vi "WPI_RobotDriveOpen2MotorWithVictor.vi"(4 "InverseTransformVIRef":T1, 5 "Right Motor Inverted":bool, 6 "TransformVIRef":T1, 7 "Left Motor Inverted":bool, 8 "error in (no error)":errorcluster, 10 "Right Motor":T5=enum."Invalid", 11 "Left Motor":T5=enum."Invalid") -> (0 "error out":errorcluster, 3 "RobotDriveDevRef":T2={"DevStatus"={"status"=FALSE, "code"=0, "source"=""}, "Motors[]"=[], "Square Inputs"=FALSE, "Max Output"=1.0, "Isochronous"=FALSE})   [LabVIEW 2011]
doc: "Opens a reference to the robot drive for a two-motor robot using Victor motor controllers.\n\nThis software is licensed. Open the labview\\readme\\WPI Robotics Library Open Source License.txt file for more information."
uses:
  <vilib>/Rock Robotics/SystemInterfaces/DIO/FPGA_DIOPWMChannel.ctl
  <vilib>/Rock Robotics/WPI/RobotDrive/WPI_RobotDriveDevRef.ctl
  <vilib>/Rock Robotics/WPI/MotorControl/WPI_MotorControlDeviceRef.ctl
  <vilib>/Rock Robotics/SystemInterfaces/Typedef/FPGA_TypedefDigitalModule.ctl
  <vilib>/Rock Robotics/WPI/PWM/WPI_PWMDeadband.ctl
  <vilib>/Rock Robotics/WPI/CAN/Jaguar/SubVIs/WPI_CANJaguar_ControlMode.ctl
  <vilib>/Rock Robotics/WPI/PWM/WPI_PWMTransform_ConPane.ctl
  <vilib>/Rock Robotics/WPI/SafetyOutput/WPI_SafetyOutputConfigMenu.ctl
  <vilib>/Rock Robotics/WPI/MotorControl/WPI_MotorControlOpen Victor.vi
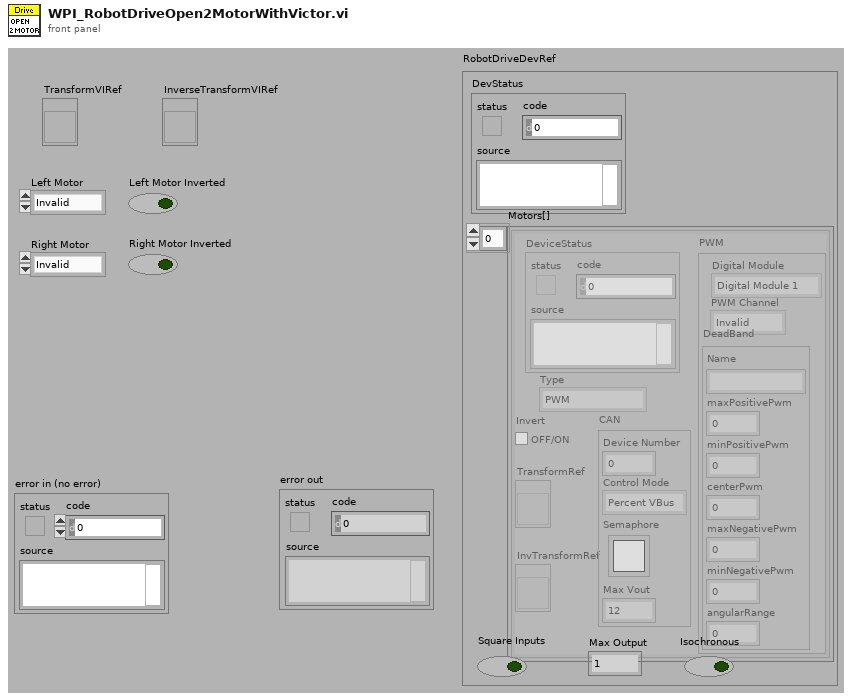
[diagram p1: front panel]
types:
  T1 = typedef "WPI_PWMTransform_ConPane.ctl" = refnum<vi>
  T2 = typedef "WPI_RobotDriveDevRef.ctl" = cluster{"DevStatus":errorcluster, "Motors[]":T3[], "Square Inputs":bool, "Max Output":dbl, "Isochronous":bool}
  T3 = typedef "WPI_MotorControlDeviceRef.ctl" = cluster{"DeviceStatus":errorcluster, "Type":enum16{"PWM", "CAN"}, "PWM":cluster{"Digital Module":T4, "PWM Channel":T5, "DeadBand":T6}, "CAN":cluster{"Device Number":u8, "Control Mode":T7, "Semaphore":T8, "Max Vout":dbl}, "Invert":bool, "TransformRef":T1, "InvTransformRef":T1}
  T4 = typedef "FPGA_TypedefDigitalModule.ctl" = enum16{"Digital Module 1", "Digital Module 2"}
  T5 = typedef "FPGA_DIOPWMChannel.ctl" = enum8{"PWM 1", "PWM 2", "PWM 3", "PWM 4", "PWM 5", "PWM 6", "PWM 7", "PWM 8", "PWM 9", "PWM 10", "Invalid"}
  T6 = typedef "WPI_PWMDeadband.ctl" = cluster{"Name":string, "maxPositivePwm":i32, "minPositivePwm":i32, "centerPwm":i32, "maxNegativePwm":i32, "minNegativePwm":i32, "angularRange":u16}
  T7 = typedef "WPI_CANJaguar_ControlMode.ctl" = enum8{"Percent VBus", "Current", "Speed", "Position", "Voltage"}
  T8 = typedef "Semaphore RefNum" = refnum<k1>
  T9 = typedef "WPI_SafetyOutputConfigMenu.ctl" = enum16{"Enable", "Disable"}
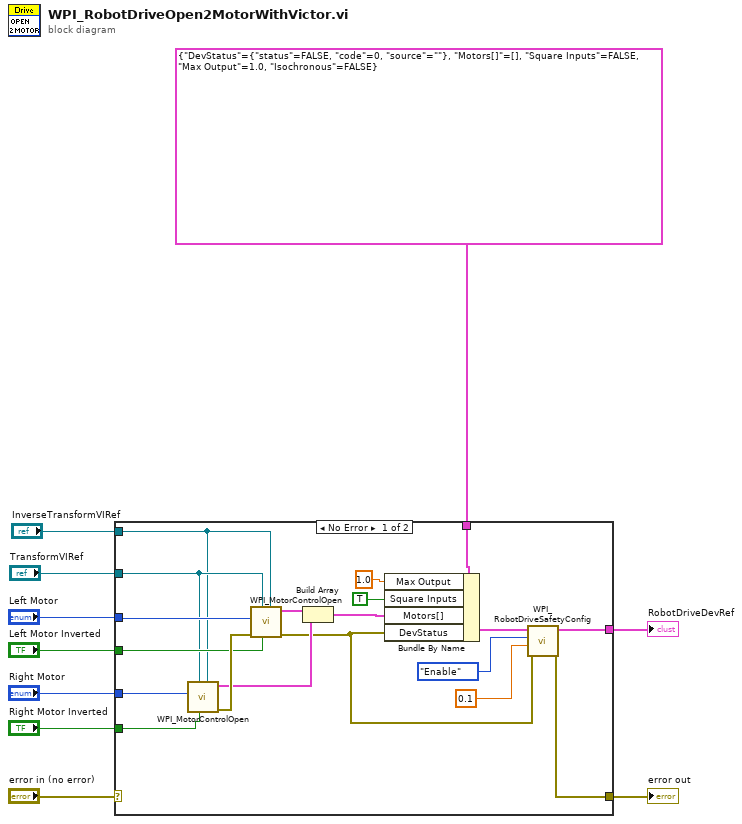
[diagram p0: block diagram]
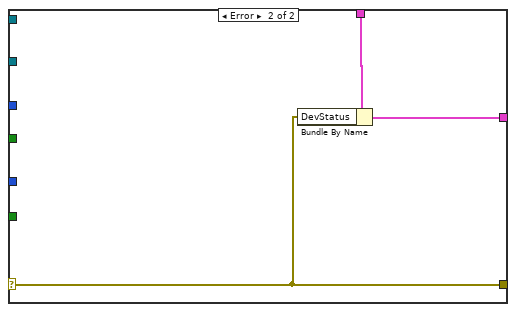
[diagram p2: hidden frame]
diagram:
  n1 = case shown="No Error" "error in (no error)" {
    selector: "error in (no error)" -> [_ w30]
    tunnel: "Left Motor" -> [w27 _]
    tunnel: "Right Motor" -> [w26 _]
    tunnel: [w15 w32] -> w3
    tunnel: "Left Motor Inverted" -> [w21 _]
    tunnel: "Right Motor Inverted" -> [w22 _]
    tunnel: T2 {"DevStatus"={"status"=FALSE, "code"=0, "source"=""}, "Motors[]"=[], "Square Inputs"=FALSE, "Max Output"=1.0, "Isochronous"=FALSE} ("RobotDriveDevRef") -> [w28 w31]
    tunnel: [w16 w30] -> w5
    tunnel: "InverseTransformVIRef" -> [w11 _]
    tunnel: "TransformVIRef" -> [w12 _]
    frame No Error {
      n2 = call-poly <vilib>:"WPI_MotorControlOpen.vi"("InverseTransformVIRef"=w11, "Invert"=w22, "TransformVIRef"=w12, "PWM Channel"=w26) -> ("error out"=w25:errorcluster, "MotorControlDeviceRef"=w23:T3)  [unwired: 3 in, 3 out]
      n3 = call-poly <vilib>:"WPI_MotorControlOpen.vi"("InverseTransformVIRef"=w11, "Invert"=w21, "TransformVIRef"=w12, "error in (no error)"=w25, "PWM Channel"=w27) -> ("error out"=w17:errorcluster, "MotorControlDeviceRef"=w24:T3)  [unwired: 2 in, 3 out]
      n4 = Build Array(w24, w23) -> (w29:T3[])
      n5 = Bundle By Name(cluster=w28, "Max Output"=1.0, "Square Inputs"=TRUE, "Motors[]"=w29, "DevStatus"=w17) -> (w19:T2)
      n6 = call <vilib>:"WPI_RobotDriveSafetyConfig.vi"("error in (no error)"=w17, "timeout (s)"=0.1, "mode"=WPI_SafetyOutputConfigMenu."Enable", "RobotDriveDevRef"=w19) -> ("error out"=w16:errorcluster, "RobotDriveDevRef"=w15:T2)  [unwired: 6 out]
    }
    frame Error {
      n7 = Bundle By Name(cluster=w31, "DevStatus"=w30) -> (w32:T2)
    }
  }
  "RobotDriveDevRef" <- w3
  "error out" <- w5
